vi "DownloadFile.vi"(8 "error in (no error)":errorcluster, 10 "Filename":string, 11 "TCP_Server_Connection_Handler in":refnum<class "TCP_Server_Connection_Handler.lvclass">) -> (0 "error out":errorcluster, 3 "TCP_Server_Connection_Handler out":refnum<class "TCP_Server_Connection_Handler.lvclass">)   [LabVIEW 2023, in "TCP_Server_Connection_Handler.lvlib" / "TCP_Server_Connection_Handler.lvclass"]
uses:
  TCP_Server_Connection_Handler.lvclass
  TCP_Server_Connection_Handler.lvclass/TCP_Server_Connection_Handler.ctl
  TCP_Server_Connection_Handler Messages/SendString Msg/SendString Msg.lvclass
  <vilib>/ActorFramework/Actor/Actor.lvclass
  <vilib>/Utility/error.llb/DialogType.ctl
  TypeDefinitions/messageType.ctl
  TCP_Server_Connection_Handler.lvlib
  C:/Program Files (x86)/National Instruments/LabVIEW 2023/vi.lib/ActorFramework/Actor/Actor.lvclass
  C:/Source/LabVIEW/TCP_server/TCP_Server_Connection_Handler/TCP_Server_Connection_Handler/TCP_Server_Connection_Handler.lvclass
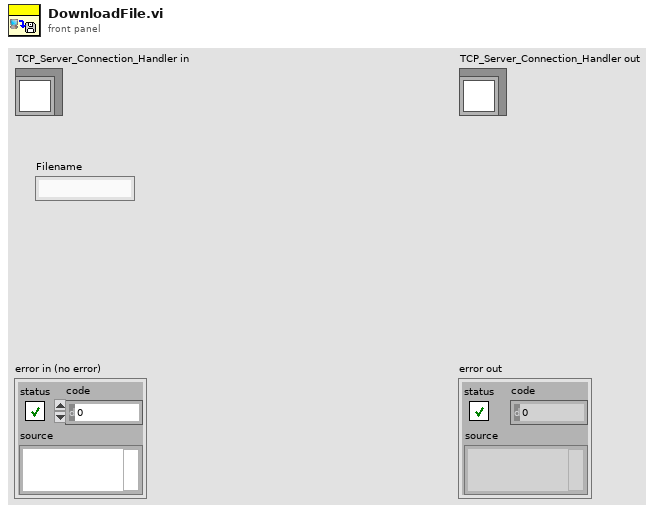
[diagram p1: front panel]
types:
  T1 = enum16{"open", "replace", "create", "open or create", "replace or create", "replace or create with confirmation"}
  T2 = typedef "TCP_Server_Connection_Handler.lvlib/messageType.ctl" = enum16{"message", "file", "get"}
  T3 = typedef "DialogType.ctl" = u16
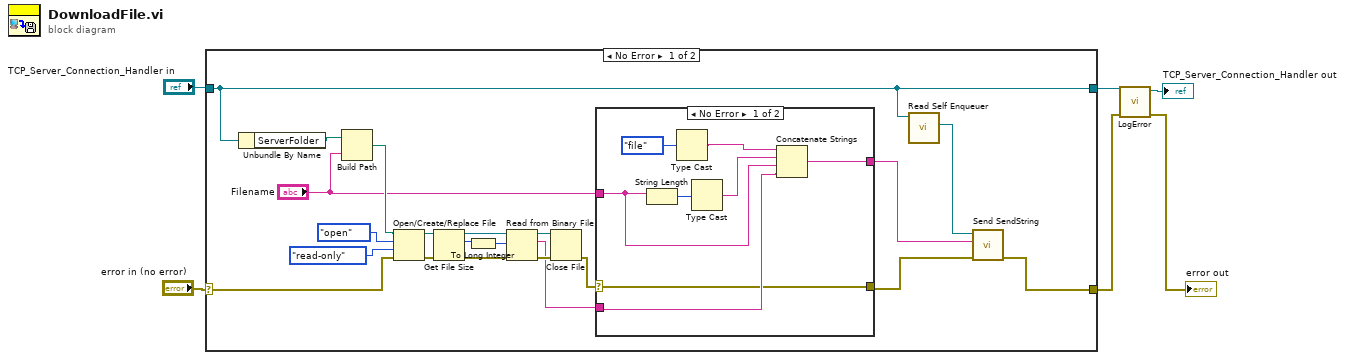
[diagram p0: block diagram]
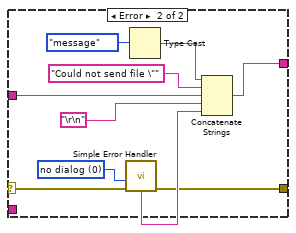
[diagram p2: hidden frame]
diagram:
  n1 = case shown="No Error" "error in (no error)" {
    selector: "error in (no error)" -> [w21 w47]
    tunnel: [w9 w47] -> w2
    tunnel: [w7 w46] -> w4
    tunnel: "TCP_Server_Connection_Handler in" -> [w7 w46]
    frame No Error {
      n2 = Unbundle By Name(w7) -> ("ServerFolder"=w27:path)
      n3 = Build Path(base path=w27, name or relative path="Filename") -> (appended path=w26:path)
      n4 = Open/Create/Replace File(file path (use dialog)=w26, error in=w21, operation (0:open)=T1."open", access (0:read/write)=enum16{"read/write", "read-only", "write-only"}."read-only") -> (refnum out=w18:refnum<file>, error out=w17:errorcluster)  [unwired: 2 in, 1 out]
      n5 = Get File Size(file=w18, error in=w17) -> (refnum out=w16:refnum<file>, size (in bytes)=w15:i64, 0:w13:errorcluster)
      n6 = To Long Integer(number=w15) -> (32bit integer=w14:i32)
      n7 = Read from Binary File(8:w13, 10:w14, 11:w16) -> (0:w23:errorcluster, 2:w11:string, 3:w22:refnum<file>)  [unwired: 3 in, 1 out]
      n8 = Close File(refnum=w22, error in=w23) -> (error out=w20:errorcluster)  [unwired: 1 out]
      n9 = case shown="No Error" w20 {
        selector: w20 -> [w28 w42]
        tunnel: "Filename" -> [w33 w44]
        tunnel: [w28 w36] -> w8
        tunnel: w11 -> [w32 _]
        tunnel: [w29 w37] -> w10
        frame No Error {
          n10 = String Length(string=w33) -> (length=w35:i32)
          n11 = Type Cast(x=messageType."file" ("MessageType")) -> (*(type *) &x=w30:string)  [unwired: 1 in]
          n12 = Type Cast(x=w35) -> (*(type *) &x=w34:string)  [unwired: 1 in]
          n13 = Concatenate Strings(w30, w34, w33, w32) -> (w29:string)
        }
        frame Error {
          w40 = T3 0 items=["no dialog", "OK message", "continue or stop message", "OK message + warnings", "continue/stop + warnings"] ("type of dialog (OK msg:1)")
          n14 = call <vilib>:"Simple Error Handler.vi"("type of dialog (OK msg:1)"=w40, "error in (no error)"=w42) -> ("error out"=w36:errorcluster, "message"=w41:string)  [unwired: 3 in, 3 out]
          n15 = Type Cast(x=messageType."message" ("MessageType")) -> (*(type *) &x=w38:string)  [unwired: 1 in]
          n16 = Concatenate Strings(w38, "Could not send file \"", w44, "\r\n", w41) -> (w37:string)
        }
      }
      n17 = call <vilib>:"Read Self Enqueuer.vi"("Actor"=w7) -> ("Self Enqueuer"=w12:refnum<class "Message Enqueuer.lvclass">)  [unwired: 10 in]
      n18 = call "Send SendString.vi"("error in (no error)"=w8, "Message"=w10, "Message Enqueuer"=w12) -> ("error out"=w9:errorcluster)  [unwired: 7 in, 1 out]
    }
    frame Error {
    }
  }
  n19 = call "LogError.vi"("error in (no error)"=w2, "TCP_Server_Connection_Handler in"=w4) -> ("error out"=→"error out":errorcluster, "TCP_Server_Connection_Handler out"=→"TCP_Server_Connection_Handler out":refnum<class "TCP_Server_Connection_Handler.lvclass">)  [unwired: 8 in]
